vi "mainModbus.vi"(8 "Error In":errorcluster, 11 "plcUDE":T1) -> (0 "Error Out":errorcluster)   [LabVIEW 2018]
uses:
  controls/modbusUDE.ctl
  controls/modbusData.ctl
  controls/readRegisterModbusCluster.ctl
  Controller Module/src/controls/controllerData.ctl
  UI Module/src/controls/mainAppElementsCluster.ctl
  Barcode Printer Module/src/controls/printData.ctl
  Barcode Scanner Module/src/controls/scanData.ctl
  controls/modbusDriverSelectorEnum.ctl
  controls/openModbusConnectionCluster.ctl
panel:
  in  "Stop":bool
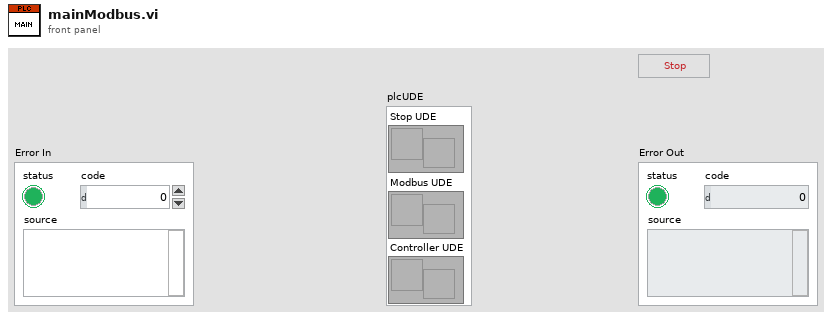
[diagram p1: front panel]
types:
  T1 = typedef "modbusUDE.ctl" = cluster{"Stop UDE":refnum<user-event>, "Modbus UDE":refnum<user-event>, "Controller UDE":refnum<user-event>}
  T2 = enum32{"Invalid", "Standard", "Closed", "Hidden", "Minimized", "Maximized"}
  T3 = enum32{"invalid app kind", "Development System", "Run Time System", "Student Edition", "Embedded LabVIEW", "Evaluation", "Custom"}
  T4 = typedef "openModbusConnectionCluster.ctl" = cluster{"IP Address":string, "Timeout (ms)":i32, "Port (502)":u16}
  T5 = typedef "modbusDriverSelectorEnum.ctl" = enum16{"open", "write single holding registers", "read holding registers", "close"}
  T6 = typedef "modbusData.ctl" = cluster{"IP Address":string, "Timeout":i32, "Port [502]":u16, "isSimulation?":bool, "Model Number":u16, "Read Modbus Register":T7, "Individual Address":u16[], "Model Changed?":bool, "Models Table":string[][], "Status?":bool}
  T7 = typedef "readRegisterModbusCluster.ctl" = cluster{"Starting Address":u16, "Number of Inputs":u16}
  T8 = cluster{"Core":cluster{"Current VI Reference":refnum<vi>, "Close Panel on Exit?":bool}, "plcUDE":T1, "Modbus Data":T6, "Registry":u16, "DB file path":path, "Models Table":string[][]}
  T9 = cluster{"Current VI Reference":refnum<vi>, "Close Panel on Exit?":bool}
  T10 = typedef "pathCluster.ctl" = cluster{"src Folder Path":path, "Controller Module Path":path, "UI Module Path":path, "Model Select Module Path":path, "Barcode Printer Module Path":path, "Barcode Scanner Module Path":path, "Database Module Path":path, "Report Generation Path":path, "Simulation Path":path, "subVIs Folder Path":path, "info Folder Path":path, "config file Path":path, "cutomerLogo Path":path, "database File Path":path}
  T11 = typedef "controllerData.ctl" = cluster{"Actions":bool[], "UI Elements Cluster":T12, "Modbus Data":T6, "Print Data":T13, "Scan Data":T14}
  T12 = typedef "mainAppElementsCluster.ctl" = cluster{"Application Name":refnum<vi>, "Tab Control":refnum<vi>, "Status":refnum<vi>, "Version No":refnum<vi>, "Result Table":refnum<vi>, "PLC":refnum<vi>, "Database":refnum<vi>, "Printer":refnum<vi>, "Scanner":refnum<vi>, "SHIFT":refnum<vi>, "OK":refnum<vi>, "NG":refnum<vi>, "TOTAL":refnum<vi>, "SCANNED BARCODE":refnum<vi>, " PRINTED BARCODE":refnum<vi>, "PART NUMBER":refnum<vi>, "PRODUCTION DATE":refnum<vi>, "SUPPLIER CODE":refnum<vi>, "SEQUENCE NUMBER":refnum<vi>, "MODEL":refnum<vi>, "Settings":refnum<vi>, "Report":refnum<vi>, "Report Table":refnum<vi>, "Home":refnum<vi>, "Export":refnum<vi>, "Fetch":refnum<vi>, "TO DATE":refnum<vi>, "FROM DATE":refnum<vi>, "Model Table":refnum<vi>, "Traceablity Graph":refnum<vi>, "Override Button":refnum<vi>, "Load Button":refnum<vi>, "Home Button-Setting":refnum<vi>, "Delete Button":refnum<vi>, "Update Button":refnum<vi>, "Save Button":refnum<vi>, "SEQUENCE NUMBER-Settings":refnum<vi>, "PLC NUMBER":refnum<vi>, "LH / RH":refnum<vi>, "SUPPLIER CODE-Setting":refnum<vi>, "CUSTOMER PART NUMBER-Setting":refnum<vi>, "MODEL-Setting":refnum<vi>, "SAVED MODEL":refnum<vi>, "NG-Settings":refnum<vi>, "OK-Settings":refnum<vi>}
  T13 = typedef "printData.ctl" = cluster{"Print Button":bool, "VISA resource name":refnum<visa-resource-name>, "Status?":bool, "Scan?":bool}
  T14 = typedef "scanData.ctl" = cluster{"Scan Button":bool, "Status?":bool}
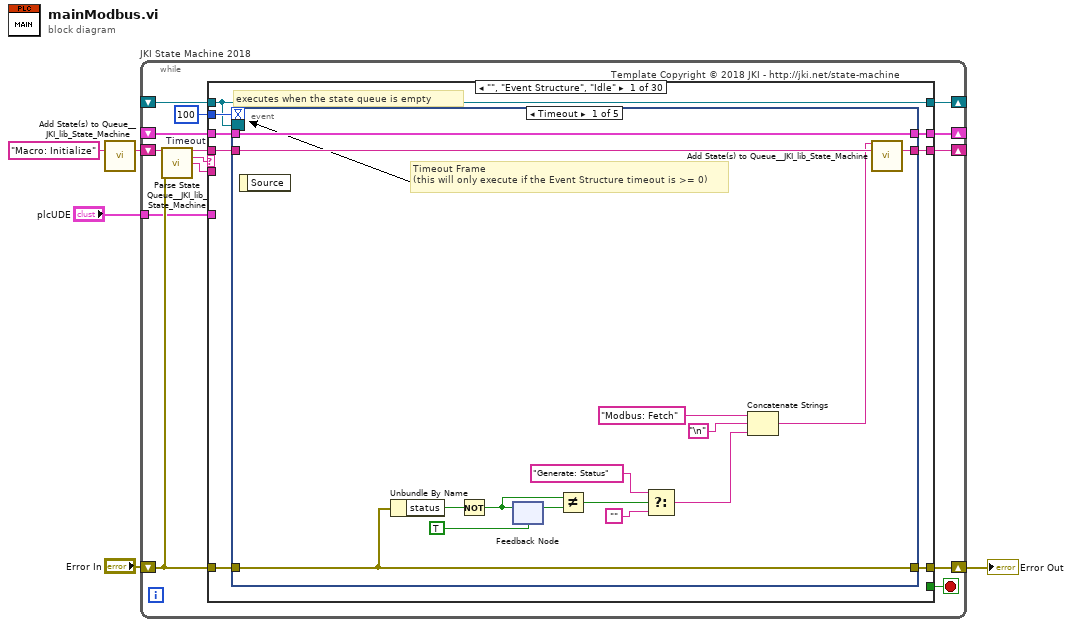
[diagram p0: block diagram]
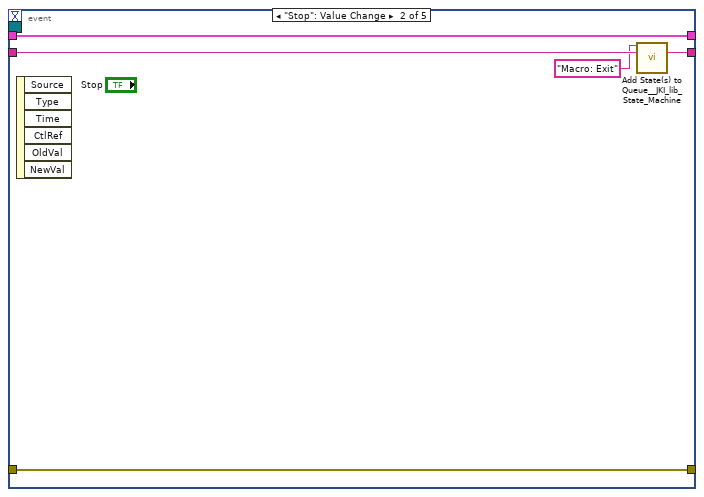
[diagram p2: hidden frame]
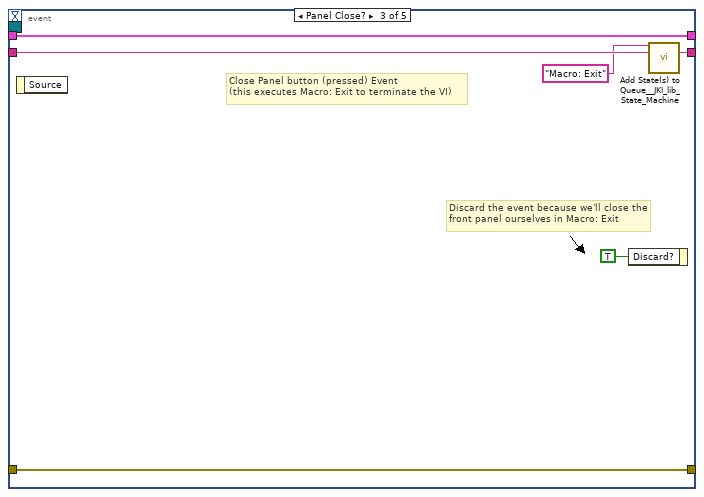
[diagram p3: hidden frame]
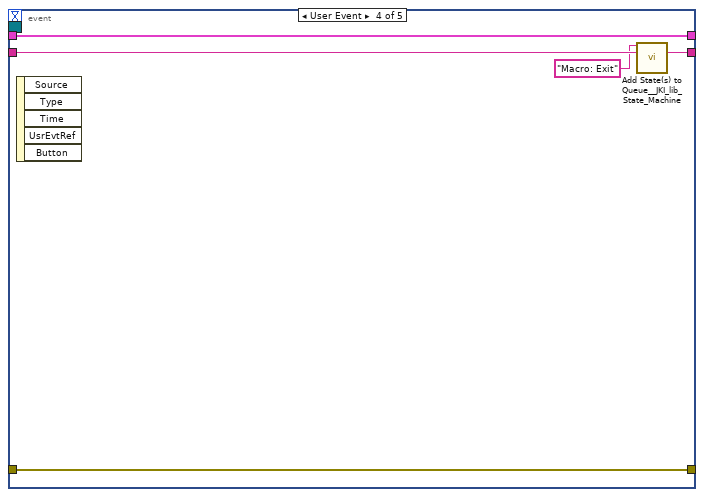
[diagram p4: hidden frame]
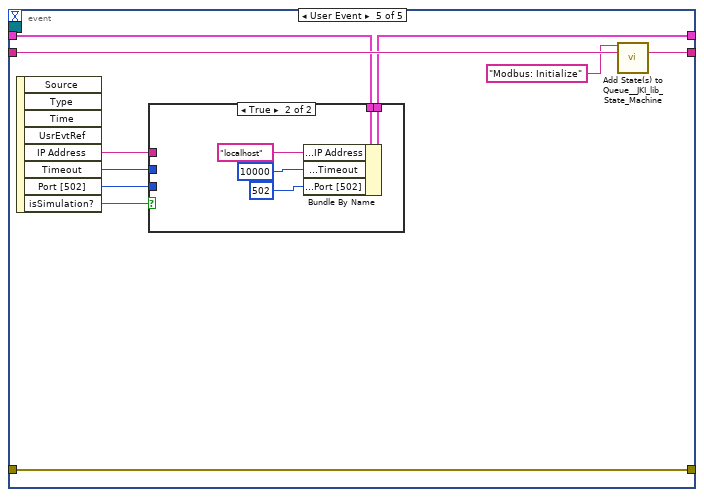
[diagram p5: hidden frame]
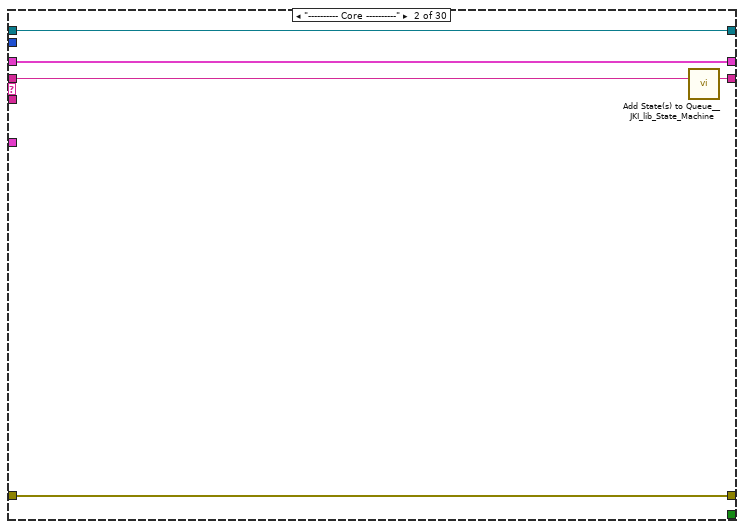
[diagram p7: hidden frame]
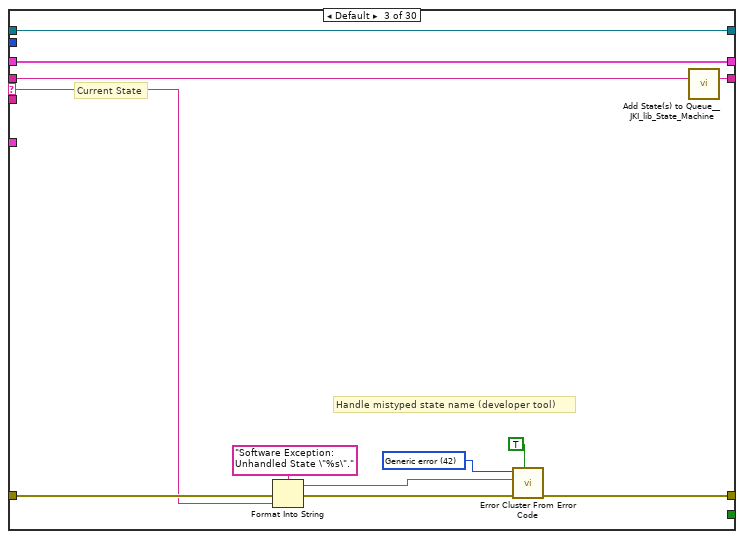
[diagram p8: hidden frame]
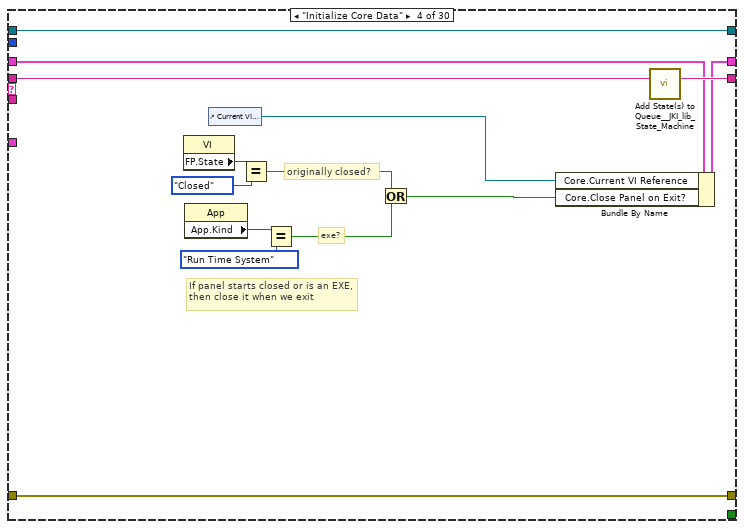
[diagram p9: hidden frame]
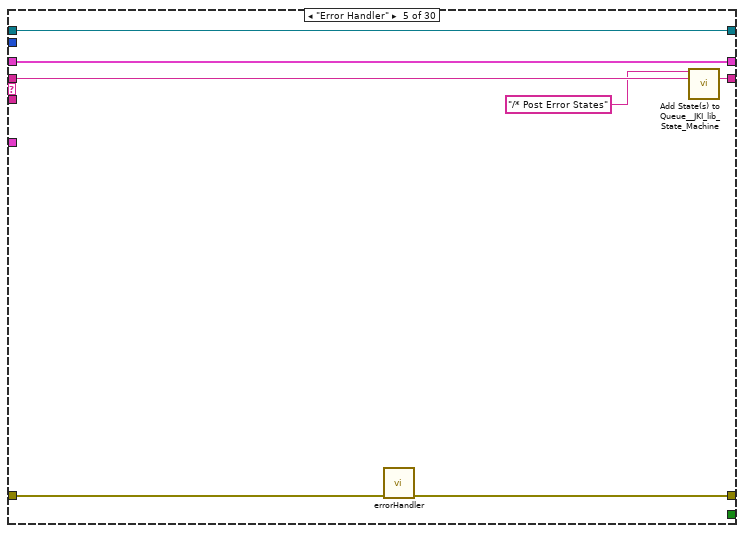
[diagram p10: hidden frame]
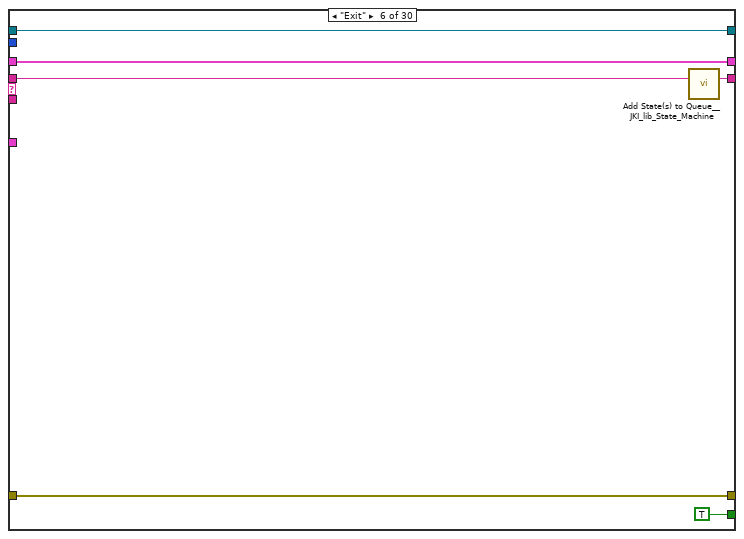
[diagram p11: hidden frame]
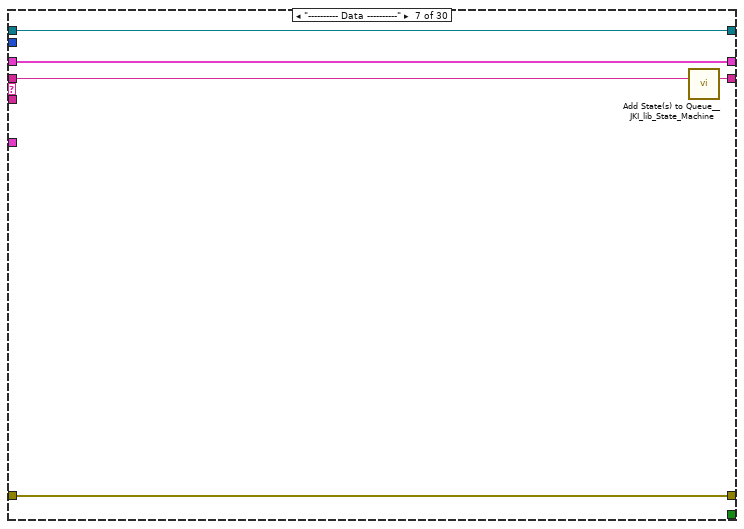
[diagram p12: hidden frame]
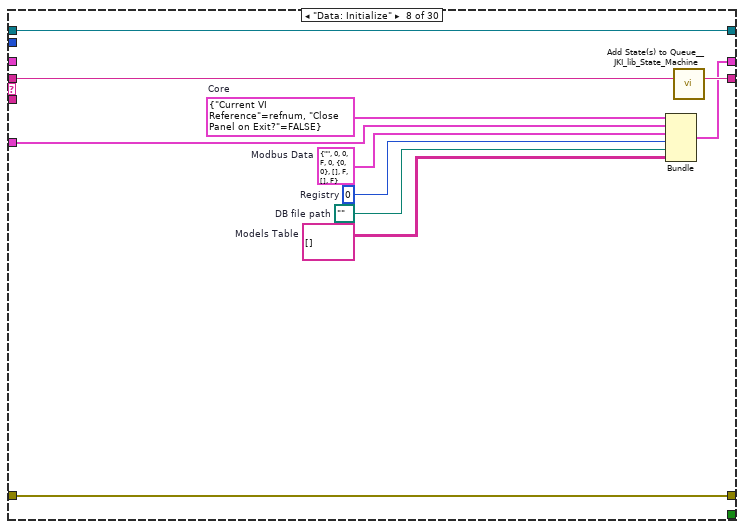
[diagram p13: hidden frame]
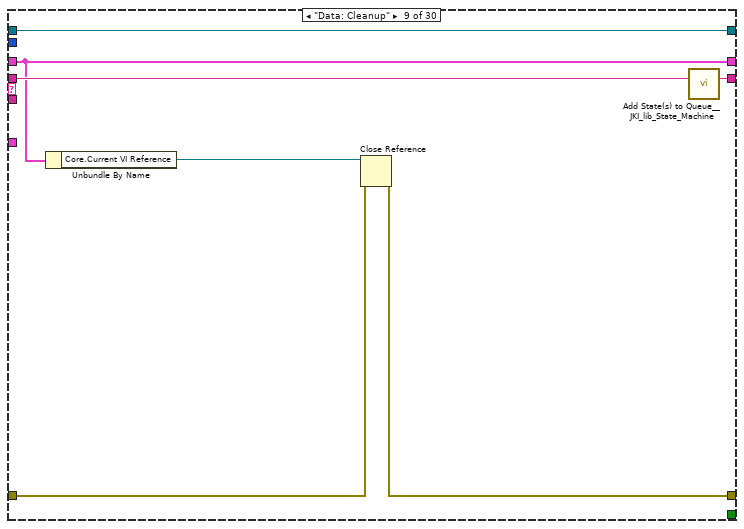
[diagram p14: hidden frame]
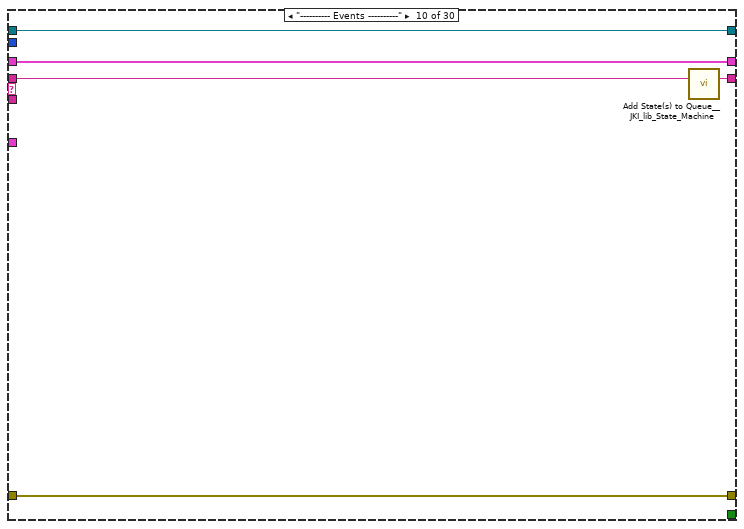
[diagram p15: hidden frame]
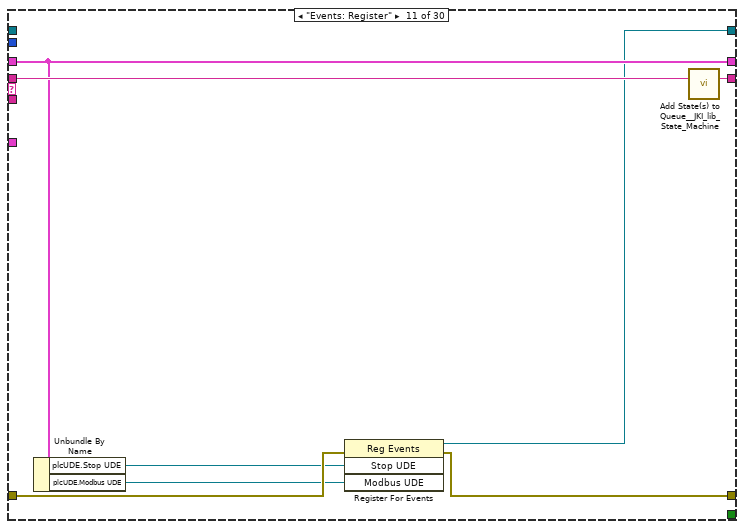
[diagram p16: hidden frame]
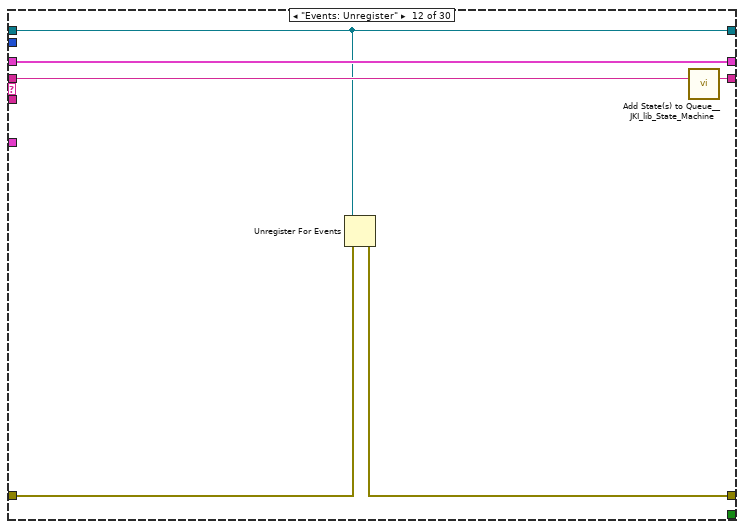
[diagram p17: hidden frame]
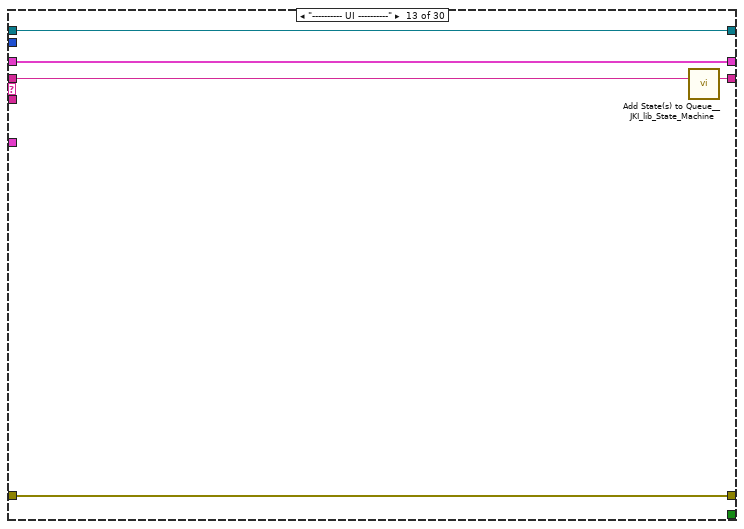
[diagram p18: hidden frame]
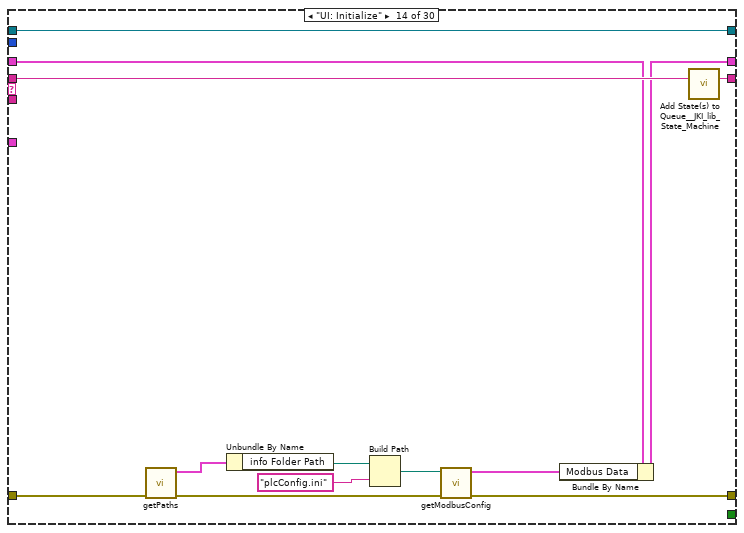
[diagram p19: hidden frame]
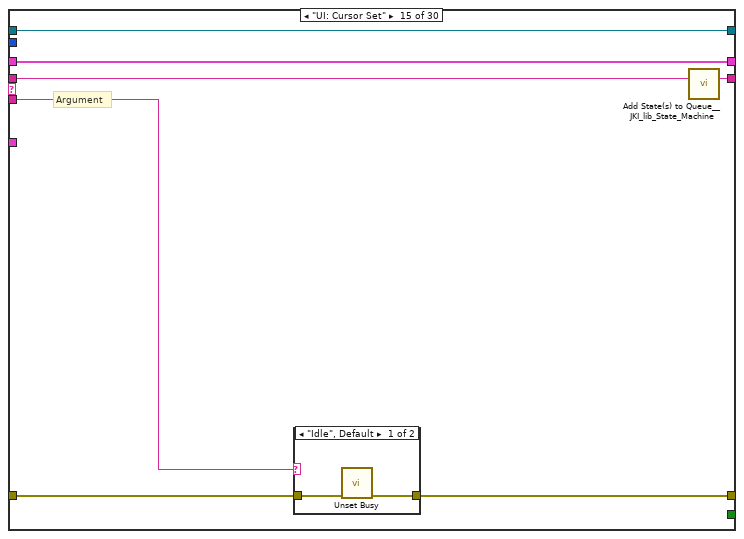
[diagram p20: hidden frame]
diagram:
  n1 = call <vilib>:"Add State(s) to Queue__JKI_lib_State_Machine.vi"("State(s) in (\"\")"="Macro: Initialize") -> ("States Out"=w5:string)  [unwired: 14 in]
  n2 = while "JKI State Machine 2018" {
    shift-right: [w12] -> _
    shift-left: _ -> [w11]
    shift-right: [w15] -> w2
    shift-left: "Error In" -> [w9]
    shift-right: [w14] -> _
    shift-left: w5 -> [w16]
    shift-right: [w8] -> _
    shift-left: _ -> [w7]
    tunnel: "plcUDE" -> [w6]
    stop <- w13 stop-if-true
    w10 = 100  # Timeout
    # "Template Copyright © 2018 JKI - http://jki.net/state-machine"
    n3 = call <vilib>:"Parse State Queue__JKI_lib_State_Machine.vi"("State Queue"=w16, "Error In (no error)"=w9) -> ("Remaining States"=w18:string, "Current State"=w19:string, "Arguments"=w17:string)  [unwired: 11 in]
    n4 = case shown="\"\", \"Event Structure\", \"Idle\"" w19 {
      selector: w19 -> [_ _ w81 _ _ _ _ _ _ _ _ _ _ _ _ _ _ _ _ _ _ _ _ _ _ _ _ _ _ _]
      tunnel: w18 -> [w27 w79 w85 w105 w112 w118 w123 w134 w141 w146 w154 w160 w165 w178 w185 w197 w267 w273 w284 w289 w305 w321 w339 w344 w349 w354 w362 w367 w375 w389]
      tunnel: w17 -> [_ _ _ _ _ _ _ _ _ _ _ _ _ _ w180 w191 _ _ _ _ _ _ _ _ _ _ _ _ _ _]
      tunnel: w11 -> [w25 w76 w83 w98 w110 w116 w120 _ w136 w143 w150 w158 w162 w168 w183 w193 w264 w270 w281 w286 w294 w311 w330 w341 w346 w351 w360 w364 w370 w384]
      tunnel: [w24 w77 w87 w102 w106 w115 w121 w131 w137 w144 w152 w155 w163 w169 w181 w194 w265 w271 w282 w287 w295 w306 w335 w340 w345 w350 w355 w365 w371 w385] -> w15
      tunnel: w9 -> [w23 w77 w86 w102 w107 w115 w121 w131 w138 w144 w151 w156 w163 w175 w182 w195 w265 w271 w282 w287 w302 w318 w336 w340 w345 w350 w358 w365 w372 w386]
      tunnel: [w26 w78 w84 w104 w111 w117 w122 w133 w140 w145 w153 w159 w164 w177 w184 w196 w266 w272 w283 w288 w304 w320 w338 w343 w348 w353 w361 w366 w374 w388] -> w14
      tunnel: [_ _ _ _ _ TRUE _ _ _ _ _ _ _ _ _ _ _ _ _ _ _ _ _ _ _ _ _ _ _ _] -> w13
      tunnel: [w22 w76 w83 w103 w110 w116 w120 w132 w136 w143 w150 w158 w162 w167 w183 w193 w264 w270 w281 w286 w293 w310 w329 w341 w346 w351 w360 w364 w370 w384] -> w12
      tunnel: w10 -> [w21 _ _ _ _ _ _ _ _ _ _ _ _ _ _ _ _ _ _ _ _ _ _ _ _ _ _ _ _ _]
      tunnel: [w20 w75 w80 w92 w108 w113 w119 w129 w135 w142 w147 w157 w161 w176 w179 w190 w263 w268 w274 w285 w303 w319 w337 w342 w347 w352 w359 w363 w373 w387] -> w8
      tunnel: w7 -> [w20 w75 w80 w92 w108 w113 w119 w129 w135 w142 _ w157 w161 w176 w179 w190 w263 w268 w274 w285 w303 w319 w337 w342 w347 w352 w359 w363 w373 w387]
      tunnel: w6 -> [_ _ _ _ _ _ _ w128 _ _ _ _ _ _ _ _ _ _ _ _ _ _ _ _ _ _ _ _ _ _]
      frame "", "Event Structure", "Idle" {
        # "executes when the state queue is empty"
        n5 = event shown="[0] Timeout" {
          selector: w20 -> [_ _ _ _ _]
          dyn-events: _ -> [_ _ _ _ _]
          timeout: w21 -> [_ _ _ _ _]
          tunnel: w27 -> [w42 w45 w53 w56 w67]
          tunnel: [w41 w44 w52 w55 w66] -> w26
          tunnel: w25 -> [w40 w47 w50 w58 w59]
          tunnel: [w36 w46 w51 w57 w68] -> w24
          tunnel: w23 -> [w36 w46 w51 w57 w68]
          tunnel: [w40 w47 w50 w58 w60] -> w22
          event Timeout {
            # "Timeout Frame\n(this will only execute if the Event Structure timeout is >= 0)"
            n6 = event-data() -> ()  [unwired: 1 in, 1 out]
            n7 = Unbundle By Name(w36) -> ("status"=w38:bool)
            n8 = Not(x=w38) -> (.not. x?=w35:bool)
            n9 = feedback #1(TRUE) -> (w39:bool)
            n10 = feedback-in #1(w35) -> ()
            n11 = Not Equal?(x=w35, y=w39) -> (x != y?=w34:bool)
            n12 = Select(t="Generate: Status" ("State(s) in Front (\"\")"), s=w34, f="") -> (s? t:f=w29:string)
            n13 = Concatenate Strings("Modbus: Fetch" ("State(s) in Front (\"\")"), "\n", w29) -> (w28:string)
            n14 = call <vilib>:"Add State(s) to Queue__JKI_lib_State_Machine.vi"("State(s) in Front (\"\")"=w28, "State(s) in (\"\")"=w42) -> ("States Out"=w41:string)  [unwired: 13 in]
          }
          event "Stop": Value Change {
            n15 = event-data() -> ()  [unwired: 1 in, 6 out]
            n16 = call <vilib>:"Add State(s) to Queue__JKI_lib_State_Machine.vi"("State(s) in Front (\"\")"="Macro: Exit" ("State(s) in Front (\"\")"), "State(s) in (\"\")"=w45) -> ("States Out"=w44:string)  [unwired: 13 in]
          }
          event Panel Close? {
            # "Discard the event because we'll close the front panel ourselves in Macro: Exit"
            # "Close Panel button (pressed) Event\n(this executes Macro: Exit to terminate the VI)"
            n17 = event-data() -> ()  [unwired: 1 in, 1 out]
            n18 = event-data("Discard?"=TRUE) -> ()  [unwired: 1 in, 1 out]
            n19 = call <vilib>:"Add State(s) to Queue__JKI_lib_State_Machine.vi"("State(s) in Front (\"\")"="Macro: Exit", "State(s) in (\"\")"=w53) -> ("States Out"=w52:string)  [unwired: 13 in]
          }
          event User Event {
            n20 = event-data() -> ()  [unwired: 1 in, 5 out]
            n21 = call <vilib>:"Add State(s) to Queue__JKI_lib_State_Machine.vi"("State(s) in Front (\"\")"="Macro: Exit" ("State(s) in Front (\"\")"), "State(s) in (\"\")"=w56) -> ("States Out"=w55:string)  [unwired: 13 in]
          }
          event User Event {
            n22 = event-data() -> ("IP Address"=w61:string, "Timeout"=w62:i32, "Port [502]"=w63:u16, "isSimulation?"=w64:bool)  [unwired: 1 in, 4 out]
            n23 = case shown="True" w64 {
              tunnel: w63 -> [_ _]
              tunnel: w62 -> [_ _]
              tunnel: w61 -> [_ _]
              tunnel: w59 -> [w69 w74]
              tunnel: [w69 w73] -> w60
              frame False {
              }
              frame True {
                n24 = Bundle By Name(cluster=w74, "Modbus Data.IP Address"="localhost" ("PLC Data.IP Address"), "Modbus Data.Timeout"=10000 ("PLC Data.Timeout"), "Modbus Data.Port [502]"=u16 502 ("PLC Data.Port [502]")) -> (w73:T8)
              }
            }
            n25 = call <vilib>:"Add State(s) to Queue__JKI_lib_State_Machine.vi"("State(s) in Front (\"\")"="Modbus: Initialize" ("State(s) in (\"\")"), "State(s) in (\"\")"=w67) -> ("States Out"=w66:string)  [unwired: 13 in]
          }
        }
      }
      frame "---------- Core ----------" {
        n26 = call <vilib>:"Add State(s) to Queue__JKI_lib_State_Machine.vi"("State(s) in (\"\")"=w79) -> ("States Out"=w78:string)  [unwired: 14 in]
      }
      frame Default {
        w90 = 42 items=["No error", "Argument error", "Memory is full", "Out of zone", "End of file", "File already open", "Generic file I/O error", "File not found", "File permission error", "Disk is full", "Duplicate path", "Too many files open", "System feature not enabled", "Resource file not found", "Cannot add resource", "Resource not found", "Image not found", "Image memory error", "Pen does not exist", "Config type invalid", "Config token not found", "Config parse error", "Config memory error", "Bad external code format", "Bad external code offset", "External code not present", "Null window", "Destroy window error", "Null menu", "Print aborted", "Bad print record", "Print driver error", "Windows error during printing", "Memory error during printing", "Print dialog error", "Generic print error", "Invalid device refnum", "Device not found", "Device parameter error", "Device unit error", "Cannot open device", "Device call aborted", "Generic error", "Cancelled by user", "Object ID too low", "Object ID too high", "Object not in heap", "Unknown heap", "Unknown object (invalid DefProc)", "Unknown object (DefProc not in table)", "Message out of range", "Invalid (null) method", "Unknown message", "Manager call not supported", "Bad address", "Network operation in progress", "Network operation timed out", "Connection is busy", "Network attribute not supported", "Network error", "Address in use", "System out of memory", "Connection aborted", "Connection refused", "Not connected", "Already connected", "Connection closed", "Initialization error (interapplication manager)", "Bad occurrence", "Wait on unbound occurrence handler", "Occurrence queue overflow", "Datalog type conflict", "Unused", "Unrecognized type (interapplication manager)", "Memory corrupt", "Failed to make temporary DLL", "Old CIN version", "Drag socket not found", "Failed to load drop-object", "Failed to register OLE object", "Failed to release OLE object", "Format specifier type mismatch", "Unknown format specifier", "Too few format specifiers", "Too many format specifiers", "Scan failed", "Newer CIN version", "Error converting to variant", "Runtime menu error", "Password tampered", "Variant attribute not found", "Incompatible variant data type", "Event data is not available", "Event Store is not present", "Occurrence is not found", "Event Queue is not created", "Event info is not available", "Refnum passed is NULL", "Error retrieving Class GUID", "Error retrieving CoClass GUID", "Error retrieving TypeLib GUID.", "Bad built application magic bytes.", "Specific driver is different from the specific driver associated with the Logical Name.", "There is no session opened to the class driver.", "Max Error", "MAX - Error with config objects", "MAX - Error loading configuration", "MAX - Group not supported"]
        # "Current State"
        # "Handle mistyped state name (developer tool)"
        n27 = Format Into String(format string="Software Exception: Unhandled State \"%s\"." ("message"), error in=w86, w81) -> (resulting string=w89:string, error out=w88:errorcluster)  [unwired: 1 in]
        n28 = call <vilib>:"Error Cluster From Error Code.vi"("show call chain? (False)"=TRUE, "error in (no error)"=w88, "error message (\"\")"=w89, "error code (0)"=w90) -> ("error out"=w87:errorcluster)  [unwired: 5 in]
        n29 = call <vilib>:"Add State(s) to Queue__JKI_lib_State_Machine.vi"("State(s) in (\"\")"=w85) -> ("States Out"=w84:string)  [unwired: 14 in]
      }
      frame "Initialize Core Data" {
        # "originally closed?"
        # "exe?"
        # "If panel starts closed or is an EXE, then close it when we exit"
        n30 = property class="VI"() -> ("FP.State"=w95:T2)  [unwired: 2 in, 2 out]
        n31 = property class="App"() -> ("App.Kind"=w101:T3)  [unwired: 2 in, 2 out]
        n32 = control-ref of="Current VI Reference"() -> (w96:refnum<vi>)
        n33 = Equal?(x=w95, y=T2."Closed" ("Front Panel Window:State")) -> (x = y?=w93:bool)
        n34 = Equal?(x=w101, y=T3."Run Time System" ("Application:Kind")) -> (x = y?=w99:bool)
        n35 = Or(x=w93, y=w99) -> (x .or. y?=w97:bool)
        n36 = Bundle By Name(cluster=w98, "Core.Current VI Reference"=w96, "Core.Close Panel on Exit?"=w97) -> (w103:T8)
        n37 = call <vilib>:"Add State(s) to Queue__JKI_lib_State_Machine.vi"("State(s) in (\"\")"=w105) -> ("States Out"=w104:string)  [unwired: 14 in]
      }
      frame "Error Handler" {
        n38 = call "errorHandler.vi"("Error In"=w107) -> ("Error Out"=w106:errorcluster)  [unwired: 10 in]
        n39 = call <vilib>:"Add State(s) to Queue__JKI_lib_State_Machine.vi"("State(s) in Front (\"\")"="/* Post Error States", "State(s) in (\"\")"=w112) -> ("States Out"=w111:string)  [unwired: 13 in]
      }
      frame "Exit" {
        n40 = call <vilib>:"Add State(s) to Queue__JKI_lib_State_Machine.vi"("State(s) in (\"\")"=w118) -> ("States Out"=w117:string)  [unwired: 14 in]
      }
      frame "---------- Data ----------" {
        n41 = call <vilib>:"Add State(s) to Queue__JKI_lib_State_Machine.vi"("State(s) in (\"\")"=w123) -> ("States Out"=w122:string)  [unwired: 14 in]
      }
      frame "Data: Initialize" {
        w124 = string[][] []  # Models Table
        w125 = path ""  # DB file path
        w126 = u16 0  # Registry
        w127 = T6 {"IP Address"="", "Timeout"=0, "Port [502]"=0, "isSimulation?"=FALSE, "Model Number"=0, "Read Modbus Register"={"Starting Address"=0, "Number of Inputs"=0}, "Individual Address"=[], "Model Changed?"=FALSE, "Models Table"=[], "Status?"=FALSE}  # Modbus Data
        w130 = T9 {"Current VI Reference"=refnum, "Close Panel on Exit?"=FALSE}  # Core
        n42 = Bundle("Core"=w130, "plcUDE"=w128, "Modbus Data"=w127, "Registry"=w126, "DB file path"=w125, "Models Table"=w124) -> (w132:T8)  [unwired: 1 in]
        n43 = call <vilib>:"Add State(s) to Queue__JKI_lib_State_Machine.vi"("State(s) in (\"\")"=w134) -> ("States Out"=w133:string)  [unwired: 14 in]
      }
      frame "Data: Cleanup" {
        n44 = Unbundle By Name(w136) -> ("Core.Current VI Reference"=w139:refnum<vi>)
        n45 = Close Reference(reference=w139, error in (no error)=w138) -> (error out=w137:errorcluster)
        n46 = call <vilib>:"Add State(s) to Queue__JKI_lib_State_Machine.vi"("State(s) in (\"\")"=w141) -> ("States Out"=w140:string)  [unwired: 14 in]
      }
      frame "---------- Events ----------" {
        n47 = call <vilib>:"Add State(s) to Queue__JKI_lib_State_Machine.vi"("State(s) in (\"\")"=w146) -> ("States Out"=w145:string)  [unwired: 14 in]
      }
      frame "Events: Register" {
        n48 = Unbundle By Name(w150) -> ("plcUDE.Stop UDE"=w149:refnum<user-event>, "plcUDE.Modbus UDE"=w148:refnum<user-event>)
        n49 = register-events(error in=w151, w149, w148) -> (reference out=w147:refnum<event-registration>, error out=w152:errorcluster)  [unwired: 1 in]
        n50 = call <vilib>:"Add State(s) to Queue__JKI_lib_State_Machine.vi"("State(s) in (\"\")"=w154) -> ("States Out"=w153:string)  [unwired: 14 in]
      }
      frame "Events: Unregister" {
        n51 = Unregister For Events(event registration refnum=w157, error in=w156) -> (error out=w155:errorcluster)
        n52 = call <vilib>:"Add State(s) to Queue__JKI_lib_State_Machine.vi"("State(s) in (\"\")"=w160) -> ("States Out"=w159:string)  [unwired: 14 in]
      }
      frame "---------- UI ----------" {
        n53 = call <vilib>:"Add State(s) to Queue__JKI_lib_State_Machine.vi"("State(s) in (\"\")"=w165) -> ("States Out"=w164:string)  [unwired: 14 in]
      }
      frame "UI: Initialize" {
        n54 = call "getPaths.vi"("Error In"=w175) -> ("Error Out"=w170:errorcluster, "Application Path Cluster"=w174:T10)  [unwired: 9 in]
        n55 = Unbundle By Name(w174) -> ("info Folder Path"=w173:path)
        n56 = Build Path(base path=w173, name or relative path="plcConfig.ini") -> (appended path=w171:path)
        n57 = call "getModbusConfig.vi"("Error In"=w170, "Modbus Config File Path"=w171) -> ("Error Out"=w169:errorcluster, "PLC Data"=w166:T6)  [unwired: 8 in]
        n58 = Bundle By Name(cluster=w168, "Modbus Data"=w166) -> (w167:T8)
        n59 = call <vilib>:"Add State(s) to Queue__JKI_lib_State_Machine.vi"("State(s) in (\"\")"=w178) -> ("States Out"=w177:string)  [unwired: 14 in]
      }
      frame "UI: Cursor Set" {
        # "Argument"
        n60 = case shown="\"Idle\", Default" w180 {
          tunnel: w182 -> [w187 w189]
          tunnel: [w186 w188] -> w181
          frame "Idle", Default {
            n61 = call <vilib>:"Unset Busy.vi"("error in (no error)"=w187) -> ("error out"=w186:errorcluster)  [unwired: 10 in]
          }
          frame "Busy" {
            n62 = call <vilib>:"Set Busy.vi"("error in (no error)"=w189) -> ("error out"=w188:errorcluster)  [unwired: 9 in, 1 out]
          }
        }
        n63 = call <vilib>:"Add State(s) to Queue__JKI_lib_State_Machine.vi"("State(s) in (\"\")"=w185) -> ("States Out"=w184:string)  [unwired: 14 in]
      }
      frame "UI: Front Panel State" {
        # "Argument"
        n64 = Unbundle By Name(w193) -> ("Core.Current VI Reference"=w192:refnum<vi>)
        n65 = case shown="\"Open\", \"Standard\", Default" w191 {
          tunnel: w195 -> [w203 w218 w229 w242 w255]
          tunnel: [w205 w219 w231 w244 w257] -> w194
          tunnel: w192 -> [w204 w216 w230 w243 w256]
          frame "Open", "Standard", Default {
            w198 = T2."Hidden" ("State")
            n66 = property class="VI"(reference=w204, error in=w203) -> (reference out=w201:refnum<vi>, error out=w202:errorcluster, "FP.State"=w200:T2)
            n67 = Not Equal?(x=w200, y=w198) -> (x != y?=w199:bool)
            n68 = case shown="True" w199 {
              tunnel: [w209 w211] -> w205
              tunnel: w202 -> [w208 w211]
              tunnel: w201 -> [w207 _]
              tunnel: w198 -> [w206 _]
              frame True {
                n69 = invoke class="VI" method="FP.Open"(reference=w207, error in=w208, "Activate"=TRUE, "State"=w206) -> (error out=w209:errorcluster)  [unwired: 1 in, 4 out]
              }
              frame False {
              }
            }
          }
          frame "Close", "Closed" {
            n70 = property class="VI"(reference=w216, error in=w218) -> (reference out=w215:refnum<vi>, error out=w217:errorcluster, "FP.State"=w213:T2)
            n71 = Not Equal?(x=w213, y=T2."Closed" ("Front Panel Window:State")) -> (x != y?=w212:bool)
            n72 = case shown="True" w212 {
              tunnel: [w220 w223] -> w219
              tunnel: w217 -> [w220 w222]
              tunnel: w215 -> [_ w221]
              frame False {
              }
              frame True {
                n73 = invoke class="VI" method="FP.Close"(reference=w221, error in=w222) -> (error out=w223:errorcluster)  [unwired: 1 in, 2 out]
              }
            }
          }
          frame "Hidden", "Hide" {
            w224 = T2."Hidden" ("State")
            n74 = property class="VI"(reference=w230, error in=w229) -> (reference out=w227:refnum<vi>, error out=w228:errorcluster, "FP.State"=w226:T2)
            n75 = Not Equal?(x=w226, y=w224) -> (x != y?=w225:bool)
            n76 = case shown="True" w225 {
              tunnel: [w235 w236] -> w231
              tunnel: w228 -> [w234 w236]
              tunnel: w227 -> [w233 _]
              tunnel: w224 -> [w232 _]
              frame True {
                n77 = invoke class="VI" method="FP.Open"(reference=w233, error in=w234, "State"=w232) -> (error out=w235:errorcluster)  [unwired: 2 in, 4 out]
              }
              frame False {
              }
            }
          }
          frame "Minimize", "Minimized" {
            w237 = T2."Minimized" ("State")
            n78 = property class="VI"(reference=w243, error in=w242) -> (reference out=w240:refnum<vi>, error out=w241:errorcluster, "FP.State"=w239:T2)
            n79 = Not Equal?(x=w239, y=w237) -> (x != y?=w238:bool)
            n80 = case shown="True" w238 {
              tunnel: [w248 w249] -> w244
              tunnel: w241 -> [w247 w249]
              tunnel: w240 -> [w246 _]
              tunnel: w237 -> [w245 _]
              frame True {
                n81 = invoke class="VI" method="FP.Open"(reference=w246, error in=w247, "State"=w245) -> (error out=w248:errorcluster)  [unwired: 2 in, 4 out]
              }
              frame False {
              }
            }
          }
          frame "Maximize", "Maximized" {
            w250 = T2."Maximized" ("State")
            n82 = property class="VI"(reference=w256, error in=w255) -> (reference out=w253:refnum<vi>, error out=w254:errorcluster, "FP.State"=w252:T2)
            n83 = Not Equal?(x=w252, y=w250) -> (x != y?=w251:bool)
            n84 = case shown="True" w251 {
              tunnel: [w261 w262] -> w257
              tunnel: w254 -> [w260 w262]
              tunnel: w253 -> [w259 _]
              tunnel: w250 -> [w258 _]
              frame True {
                n85 = invoke class="VI" method="FP.Open"(reference=w259, error in=w260, "State"=w258) -> (error out=w261:errorcluster)  [unwired: 2 in, 4 out]
              }
              frame False {
              }
            }
          }
        }
        n86 = call <vilib>:"Add State(s) to Queue__JKI_lib_State_Machine.vi"("State(s) in (\"\")"=w197) -> ("States Out"=w196:string)  [unwired: 14 in]
      }
      frame "---------- Macro ----------" {
        n87 = call <vilib>:"Add State(s) to Queue__JKI_lib_State_Machine.vi"("State(s) in (\"\")"=w267) -> ("States Out"=w266:string)  [unwired: 14 in]
      }
      frame "Macro: Initialize" {
        n88 = call <vilib>:"Add State(s) to Queue__JKI_lib_State_Machine.vi"("State(s) in Front (\"\")"="Data: Initialize\nInitialize Core Data\nEvents: Register\nUI: Initialize\nModbus: Initialize\nUI: Front Panel State >> Open", "State(s) in (\"\")"=w273) -> ("States Out"=w272:string)  [unwired: 13 in]
      }
      frame "Macro: Exit" {
        n89 = Unbundle By Name(w281) -> ("Core.Close Panel on Exit?"=w280:bool)
        n90 = Select(t="UI: Front Panel State >> Close", s=w280, f="") -> (s? t:f=w277:string)
        n91 = call <vilib>:"Add State(s) to Queue__JKI_lib_State_Machine.vi"("State(s) in (\"\")"=w277, "State(s) at Back (\"\")"="Modbus: Close\nData: Cleanup\nEvents: Unregister\nExit") -> ("States Out"=w275:string)  [unwired: 13 in]
        n92 = call <vilib>:"Add State(s) to Queue__JKI_lib_State_Machine.vi"("State(s) in Front (\"\")"=w275, "State(s) in (\"\")"=w284) -> ("States Out"=w283:string)  [unwired: 13 in]
      }
      frame "---------- Modbus ----------" {
        n93 = call <vilib>:"Add State(s) to Queue__JKI_lib_State_Machine.vi"("State(s) in (\"\")"=w289) -> ("States Out"=w288:string)  [unwired: 14 in]
      }
      frame "Modbus: Initialize" {
        n94 = Unbundle By Name(w294) -> ("Modbus Data.IP Address"=w298:string, "Modbus Data.Timeout"=w296:i32, "Modbus Data.Port [502]"=w297:u16)
        n95 = Bundle By Name(cluster=T4 {"IP Address"="", "Timeout (ms)"=0, "Port (502)"=0} ("Open Modbus Connection Cluster"), "IP Address"=w298, "Timeout (ms)"=w296, "Port (502)"=w297) -> (w299:T4)
        n96 = call "modbusTCPMasterDriver.vi"("Modbus Driver Selector Enum"=modbusDriverSelectorEnum."open", "Error In"=w302, "Open Modbus Connection Cluster"=w299) -> ("Error Out"=w295:errorcluster)  [unwired: 7 in, 1 out]
        n97 = Unbundle By Name(w295) -> ("status"=w292:bool)
        n98 = Not(x=w292) -> (.not. x?=w290:bool)
        n99 = Bundle By Name(cluster=w294, "Modbus Data.Status?"=w290) -> (w293:T8)
        n100 = call <vilib>:"Add State(s) to Queue__JKI_lib_State_Machine.vi"("State(s) in Front (\"\")"="Generate: Status" ("State(s) in Front (\"\")"), "State(s) in (\"\")"=w305) -> ("States Out"=w304:string)  [unwired: 13 in]
      }
      frame "Modbus: Fetch" {
        n101 = Unbundle By Name(w311) -> ("Modbus Data.Read Modbus Register"=w316:T7)
        n102 = call "modbusTCPMasterDriver.vi"("Modbus Driver Selector Enum"=modbusDriverSelectorEnum."read holding registers", "Error In"=w318, "Read Modbus Register"=w316) -> ("Error Out"=w306:errorcluster, "Register Value"=w309:u16[])  [unwired: 7 in]
        n103 = feedback #2() -> (w314:u16[])  [unwired: 1 in]
        n104 = feedback-in #2(w309) -> ()
        n105 = Not Equal?(x=w309, y=w314) -> (x != y?=w315:bool[])
        n106 = Search 1D Array(1D array=w315, element=TRUE) -> (index of element=w308:i32)  [unwired: 1 in]
        n107 = case shown="-1, Default" w308 {
          tunnel: ["" "Modbus: Model" "Modbus: Print" "Modbus: Cycle start" "Modbus: Cycle End"] -> w312
          frame -1, Default {
          }
          frame 0 {
          }
          frame 1 {
          }
          frame 3 {
          }
          frame 4 {
          }
        }
        n108 = Index Array(array=w309, index=w308) -> (element=w307:u16)
        n109 = Bundle By Name(cluster=w311, "Registry"=w307) -> (w310:T8)
        n110 = call <vilib>:"Add State(s) to Queue__JKI_lib_State_Machine.vi"("State(s) in Front (\"\")"=w312, "State(s) in (\"\")"=w321) -> ("States Out"=w320:string)  [unwired: 13 in]
      }
      frame "Modbus: Model" {
        # "SELECT *\nFROM MODEL\nWHERE plcNumber = '34';"
        n111 = Unbundle By Name(w330) -> ("Registry"=w332:u16)
        n112 = Number To Decimal String(number=w332) -> (decimal integer string=w331:string)  [unwired: 1 in]
        n113 = Concatenate Strings("SELECT *\nFROM MODEL\nWHERE plcNumber = '" ("string"), w331, "';") -> (w334:string)
        n114 = call "queryAndFetch.vi"("Error In"=w336, "Query"=w334) -> ("Error Out"=w335:errorcluster, "Result Table"=w328:string[][])  [unwired: 8 in]
        n115 = Bundle By Name(cluster=w330, "Models Table"=w328) -> (w329:T8)
        n116 = call <vilib>:"Add State(s) to Queue__JKI_lib_State_Machine.vi"("State(s) in (\"\")"=w339) -> ("States Out"=w338:string)  [unwired: 14 in]
      }
      frame "Modbus: Print" {
        n117 = Unbundle By Name(w341) -> ()  [unwired: 1 out]
        n118 = call <vilib>:"Add State(s) to Queue__JKI_lib_State_Machine.vi"("State(s) in (\"\")"=w344) -> ("States Out"=w343:string)  [unwired: 14 in]
      }
      frame "Modbus: Cycle start" {
        n119 = Unbundle By Name(w346) -> ()  [unwired: 1 out]
        n120 = call <vilib>:"Add State(s) to Queue__JKI_lib_State_Machine.vi"("State(s) in (\"\")"=w349) -> ("States Out"=w348:string)  [unwired: 14 in]
      }
      frame "Modbus: Cycle End" {
        n121 = Unbundle By Name(w351) -> ()  [unwired: 1 out]
        n122 = call <vilib>:"Add State(s) to Queue__JKI_lib_State_Machine.vi"("State(s) in (\"\")"=w354) -> ("States Out"=w353:string)  [unwired: 14 in]
      }
      frame "Modbus: Close" {
        n123 = call "modbusTCPMasterDriver.vi"("Modbus Driver Selector Enum"=modbusDriverSelectorEnum."close", "Error In"=w358) -> ("Error Out"=w356:errorcluster)  [unwired: 8 in, 1 out]
        n124 = call <vilib>:"Clear Errors.vi"("error in (no error)"=w356) -> ("error out"=w355:errorcluster)  [unwired: 5 in, 1 out]
        n125 = call <vilib>:"Add State(s) to Queue__JKI_lib_State_Machine.vi"("State(s) in (\"\")"=w362) -> ("States Out"=w361:string)  [unwired: 14 in]
      }
      frame "---------- Generate ----------" {
        n126 = call <vilib>:"Add State(s) to Queue__JKI_lib_State_Machine.vi"("State(s) in (\"\")"=w367) -> ("States Out"=w366:string)  [unwired: 14 in]
      }
      frame "Generate: Status" {
        n127 = Unbundle By Name(w370) -> ("plcUDE.Modbus UDE"=w369:refnum<user-event>, "Modbus Data"=w368:T6)
        n128 = Generate User Event(user event=w369, event data cluster=w368, error in=w372) -> (error out=w371:errorcluster)  [unwired: 1 in, 1 out]
        n129 = call <vilib>:"Add State(s) to Queue__JKI_lib_State_Machine.vi"("State(s) in (\"\")"=w375) -> ("States Out"=w374:string)  [unwired: 14 in]
      }
      frame "Generate: Model Change" {
        w379 = T11 {"Actions"=[], "UI Elements Cluster"={"Application Name"=refnum, "Tab Control"=refnum, "Status"=refnum, "Version No"=refnum, "Result Table"=refnum, "PLC"=refnum, "Database"=refnum, "Printer"=refnum, "Scanner"=refnum, "SHIFT"=refnum, "OK"=refnum, "NG"=refnum, "TOTAL"=refnum, "SCANNED BARCODE"=refnum, " PRINTED BARCODE"=refnum, "PART NUMBER"=refnum, "PRODUCTION DATE"=refnum, "SUPPLIER CODE"=refnum, "SEQUENCE NUMBER"=refnum, "MODEL"=refnum, "Settings"=refnum, "Report"=refnum, "Report Table"=refnum, "Home"=refnum, "Export"=refnum, "Fetch"=refnum, "TO DATE"=refnum, "FROM DATE"=refnum, "Model Table"=refnum, "Traceablity Graph"=refnum, "Override Button"=refnum, "Load Button"=refnum, "Home Button-Setting"=refnum, "Delete Button"=refnum, "Update Button"=refnum, "Save Button"=refnum, "SEQUENCE NUMBER-Settings"=refnum, "PLC NUMBER"=refnum, "LH / RH"=refnum, "SUPPLIER CODE-Setting"=refnum, "CUSTOMER PART NUMBER-Setting"=refnum, "MODEL-Setting"=refnum, "SAVED MODEL"=refnum, "NG-Settings"=refnum, "OK-Settings"=refnum}, "Modbus Data"={"IP Address"="", "Timeout"=0, "Port [502]"=0, "isSimulation?"=FALSE, "Model Number"=0, "Read Modbus Register"={"Starting Address"=0, "Number of Inputs"=1}, "Individual Address"=[], "Model Changed?"=FALSE, "Models Table"=[], "Status?"=FALSE}, "Print Data"={"Print Button"=FALSE, "VISA resource name"="", "Status?"=FALSE, "Scan?"=FALSE}, "Scan Data"={"Scan Button"=FALSE, "Status?"=FALSE}} ("event data")
        n130 = Unbundle By Name(w384) -> ("Models Table"=w381:string[][], "plcUDE.Controller UDE"=w383:refnum<user-event>)
        n131 = Unbundle By Name(w379) -> ("Actions"=w378:bool[])
        n132 = Insert Into Array(array=w378, index=21, new element=TRUE ("new element/subarray")) -> (w380:bool[])
        n133 = Bundle By Name(cluster=w379, "Actions"=w380, "Modbus Data.Models Table"=w381) -> (w382:T11)
        n134 = Generate User Event(user event=w383, event data cluster=w382, error in=w386) -> (error out=w385:errorcluster)  [unwired: 1 in, 1 out]
        n135 = call <vilib>:"Add State(s) to Queue__JKI_lib_State_Machine.vi"("State(s) in (\"\")"=w389) -> ("States Out"=w388:string)  [unwired: 14 in]
      }
    }
  }
  "Error Out" <- w2
